vi "RTS Get TDMS Data.vi"(0 "CSV Data Save":T2, 1 "Chamber 1 Socket":string[][](array[string]), 2 "Chamber 2 Socket":string[][](array[string]), 3 "Chamber 3 Socket":string[][](array[string]), 4 "Chamber 4 Socket":string[][](array[string]), 5 "error in (no error)":errorcluster, 9 "Tree Selection":T1) -> (14 "Station Data":dbl[][](array[numeric]), 15 "Point File Name":string, 19 "error out":errorcluster)   [LabVIEW 2016]
uses:
  Type Definitions/RTS TDMS Filename Locations.ctl
  Type Definitions/RTS Save References.ctl
  Type Definitions/RTS Room Selector.ctl
  Type Definitions/RTS TDMS Data.ctl
panel:
  out "Indexed Full Names":string[](array[string])
  out "Index Locations":i32[](array[numeric])
  out "Custom Titles":string[](array[string])
  out "Item Names":string[](array[string])
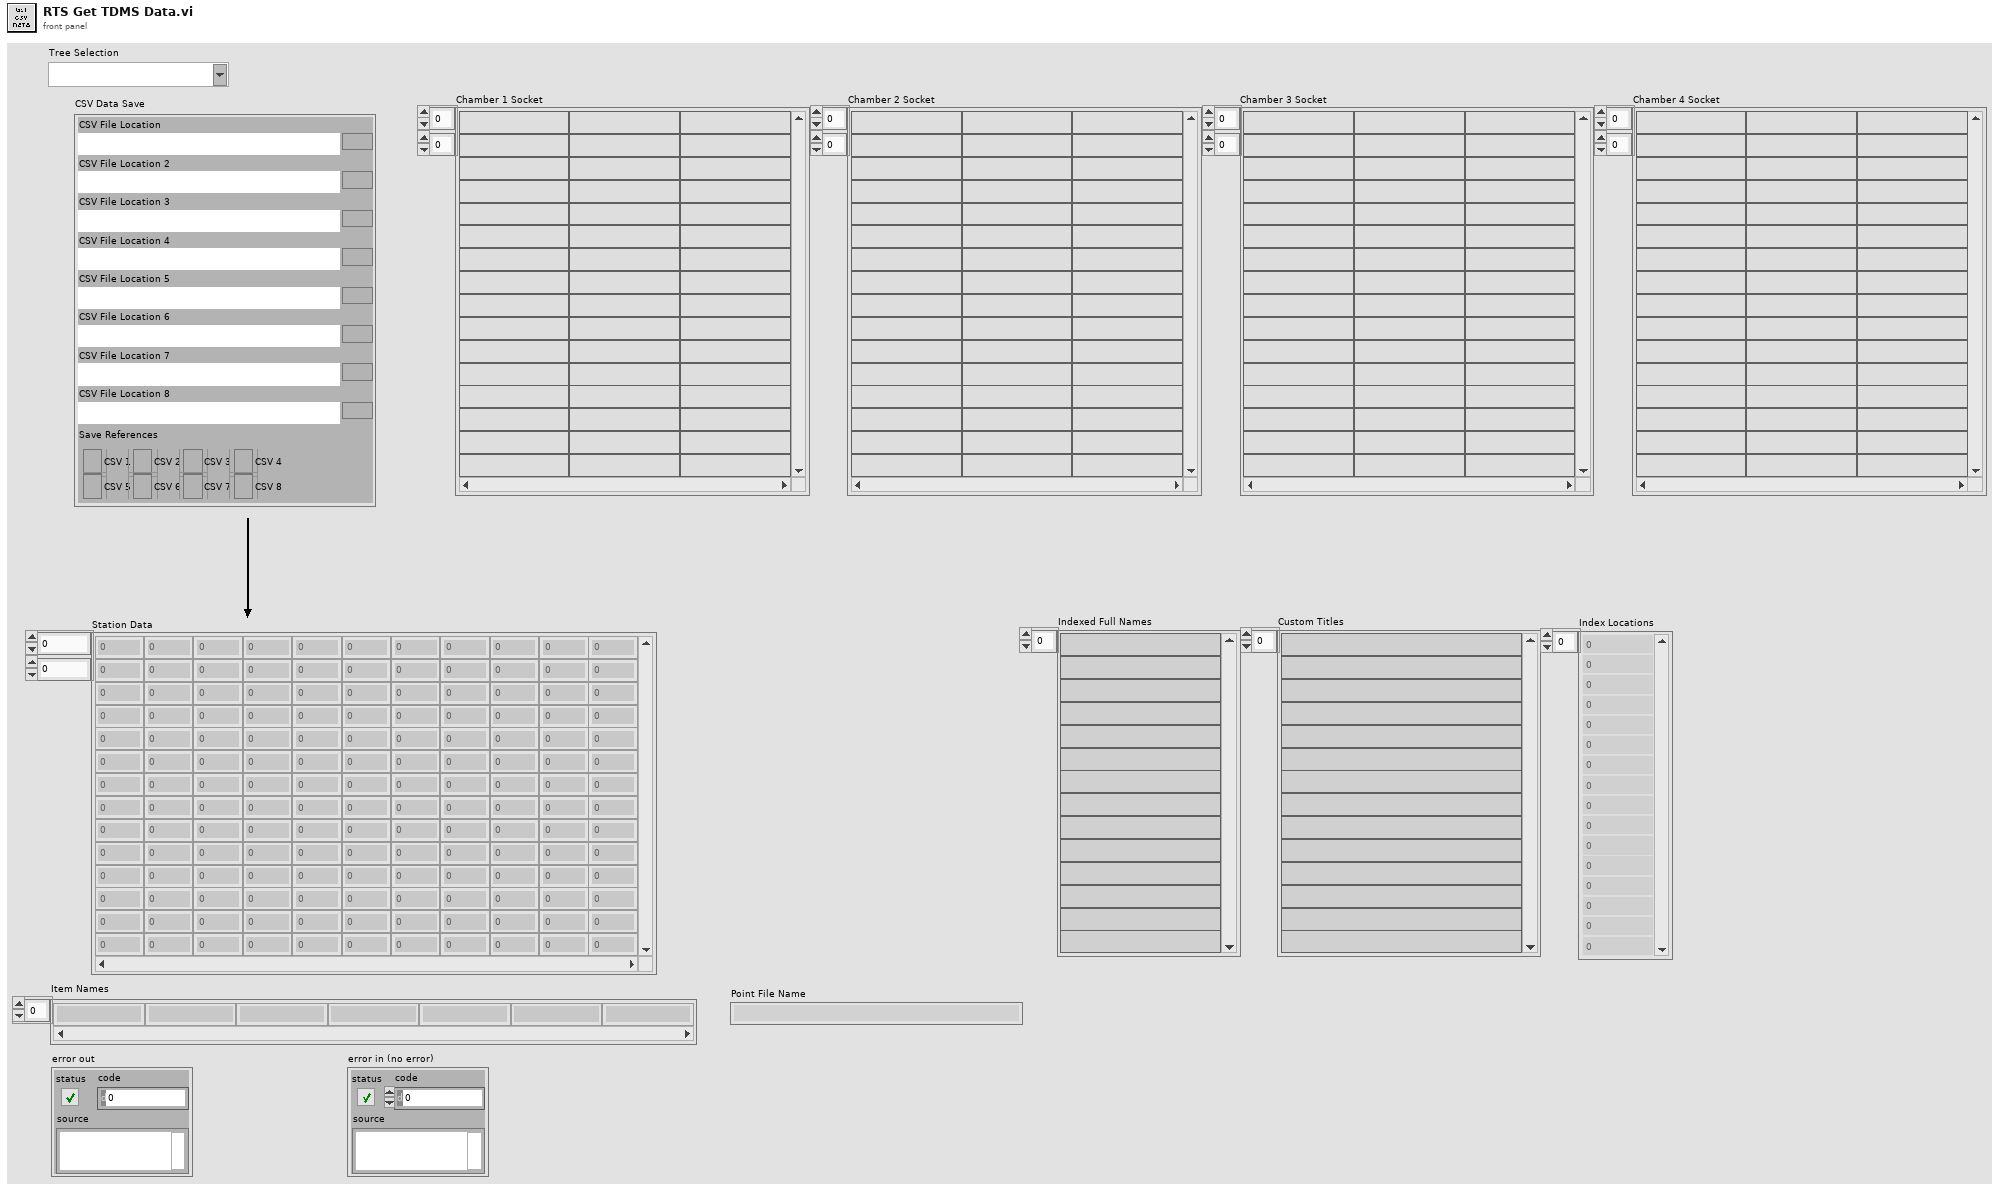
[diagram p1: front panel]
types:
  T1 = typedef "RTS Room Selector.ctl" = string
  T2 = typedef "RTS TDMS Filename Locations.ctl" = cluster{"CSV File Location":path, "CSV File Location 2":path, "CSV File Location 3":path, "CSV File Location 4":path, "CSV File Location 5":path, "CSV File Location 6":path, "CSV File Location 7":path, "CSV File Location 8":path, "Save References":T3}
  T3 = typedef "RTS Save References.ctl" = cluster{"CSV 1":refnum<file>, "CSV 2":refnum<file>, "CSV 3":refnum<file>, "CSV 4":refnum<file>, "CSV 5":refnum<file>, "CSV 6":refnum<file>, "CSV 7":refnum<file>, "CSV 8":refnum<file>}
  T4 = typedef "RTS TDMS Data.ctl" = cluster{"Station 1":dbl[][], "Station 2":dbl[][], "Station 3":dbl[][], "Station 4":dbl[][], "Station 5":dbl[][], "Station 6":dbl[][], "Station 7":dbl[][], "Station 8":dbl[][]}
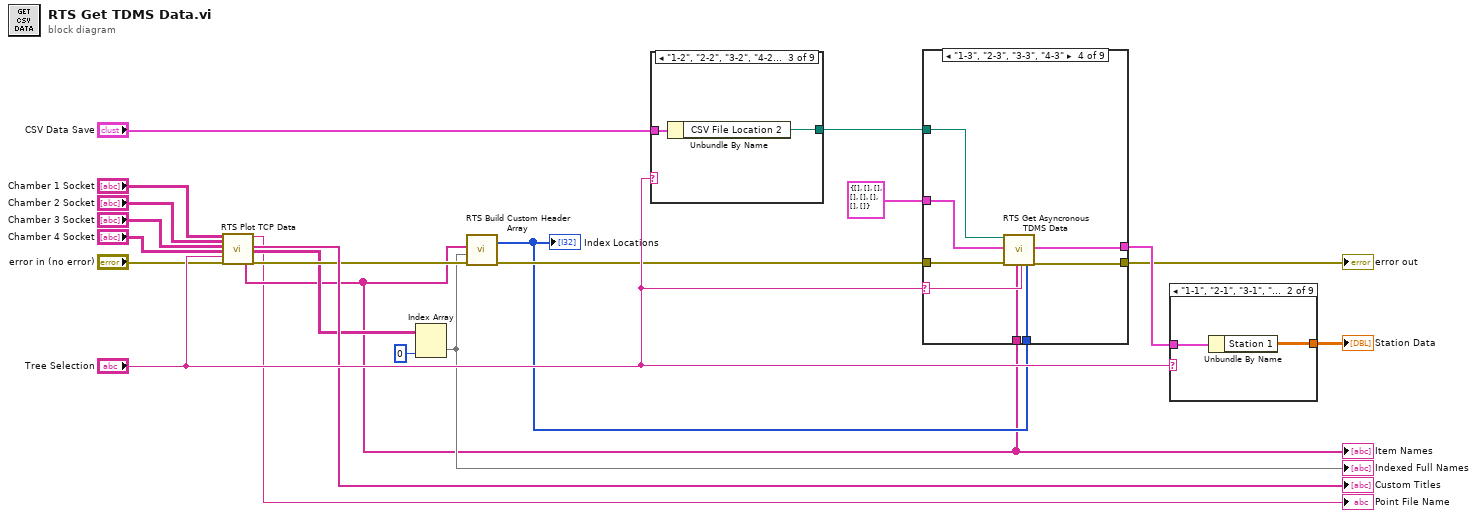
[diagram p0: block diagram]
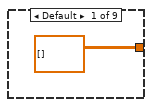
[diagram p2: hidden frame]
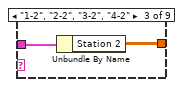
[diagram p3: hidden frame]
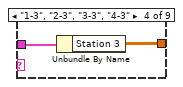
[diagram p4: hidden frame]
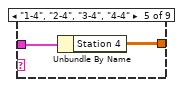
[diagram p5: hidden frame]
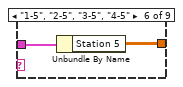
[diagram p6: hidden frame]
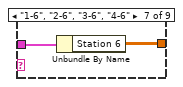
[diagram p7: hidden frame]
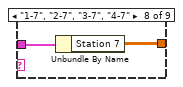
[diagram p8: hidden frame]
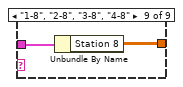
[diagram p9: hidden frame]
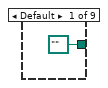
[diagram p10: hidden frame]
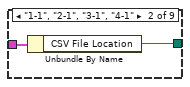
[diagram p11: hidden frame]
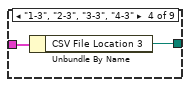
[diagram p12: hidden frame]
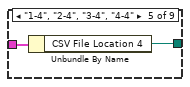
[diagram p13: hidden frame]
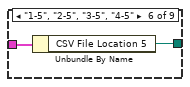
[diagram p14: hidden frame]
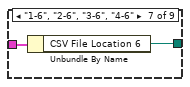
[diagram p15: hidden frame]
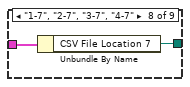
[diagram p16: hidden frame]
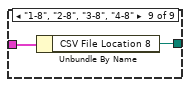
[diagram p17: hidden frame]
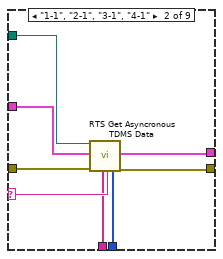
[diagram p19: hidden frame]
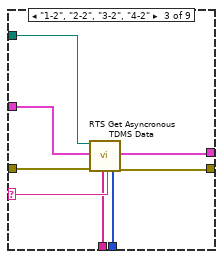
[diagram p20: hidden frame]
diagram:
  n1 = call "RTS Plot TCP Data.vi"("Chamber 1 Socket"="Chamber 1 Socket", "Chamber 2 Socket"="Chamber 2 Socket", "Chamber 3 Socket"="Chamber 3 Socket", "Chamber 4 Socket"="Chamber 4 Socket", "Tree Selection in"="Tree Selection", "Error In"="error in (no error)") -> ("Full Item Names"=w3:string[], "Point File Name"=→"Point File Name":string, "Custom Titles"=→"Custom Titles":string[], "Listbox Data"=w11:string[][], "Error Out"=w13:errorcluster)  [unwired: 6 in, 3 out]
  "Item Names" <- w3
  n2 = Index Array(array=w11, index (col)=0 ("disabled index (col)")) -> (element=w9:string[])  [unwired: 1 in]
  "Indexed Full Names" <- w9
  n3 = call "RTS Build Custom Header Array.vi"("Error In"=w13, "Listbox Item Names in"=w9, "Full Item Names"=w3) -> ("Error Out"=w12:errorcluster, "Index Locations"=w4:i32[])  [unwired: 4 in, 3 out]
  "Index Locations" <- w4
  n4 = case shown="\"1-2\", \"2-2\", \"3-2\", \"4-2\"" "Tree Selection" {
    tunnel: "CSV Data Save" -> [_ w24 w26 w28 w30 w32 w34 w36 w38]
    tunnel: [path "" ("CSV File Location 7") w23 w25 w27 w29 w31 w33 w35 w37] -> w7
    frame Default {
    }
    frame "1-1", "2-1", "3-1", "4-1" {
      n5 = Unbundle By Name(w24) -> ("CSV File Location"=w23:path)
    }
    frame "1-2", "2-2", "3-2", "4-2" {
      n6 = Unbundle By Name(w26) -> ("CSV File Location 2"=w25:path)
    }
    frame "1-3", "2-3", "3-3", "4-3" {
      n7 = Unbundle By Name(w28) -> ("CSV File Location 3"=w27:path)
    }
    frame "1-4", "2-4", "3-4", "4-4" {
      n8 = Unbundle By Name(w30) -> ("CSV File Location 4"=w29:path)
    }
    frame "1-5", "2-5", "3-5", "4-5" {
      n9 = Unbundle By Name(w32) -> ("CSV File Location 5"=w31:path)
    }
    frame "1-6", "2-6", "3-6", "4-6" {
      n10 = Unbundle By Name(w34) -> ("CSV File Location 6"=w33:path)
    }
    frame "1-7", "2-7", "3-7", "4-7" {
      n11 = Unbundle By Name(w36) -> ("CSV File Location 7"=w35:path)
    }
    frame "1-8", "2-8", "3-8", "4-8" {
      n12 = Unbundle By Name(w38) -> ("CSV File Location 8"=w37:path)
    }
  }
  n13 = case shown="\"1-3\", \"2-3\", \"3-3\", \"4-3\"" "Tree Selection" {
    selector: "Tree Selection" -> [_ w43 w51 w59 w67 w76 w85 w92 w101]
    tunnel: T4 {"Station 1"=[], "Station 2"=[], "Station 3"=[], "Station 4"=[], "Station 5"=[], "Station 6"=[], "Station 7"=[], "Station 8"=[]} ("CSV Data") -> [w39 w48 w54 w62 w70 w79 w87 w95 w99]
    tunnel: [w39 w47 w55 w63 w71 w75 w83 w91 w104] -> w6
    tunnel: w7 -> [_ w46 w56 w64 w72 w80 w88 w96 w100]
    tunnel: w12 -> [w40 w45 w53 w61 w69 w78 w86 w94 w102]
    tunnel: [w40 w44 w52 w60 w68 w77 w84 w93 w103] -> w1
    tunnel: w4 -> [_ w42 w49 w57 w65 w73 w81 w89 w97]
    tunnel: w3 -> [_ w41 w50 w58 w66 w74 w82 w90 w98]
    frame Default {
    }
    frame "1-1", "2-1", "3-1", "4-1" {
      n14 = call "RTS Get Asyncronous TDMS Data.vi"("File Location"=w46, "CVS Data Input"=w48, "error in (no error)"=w45, "Full Item Names"=w41, "Station ID"=w43, "Index Locations"=w42) -> ("CVS Data Output"=w47:T4, "error out"=w44:errorcluster)  [unwired: 12 in]
    }
    frame "1-2", "2-2", "3-2", "4-2" {
      n15 = call "RTS Get Asyncronous TDMS Data.vi"("File Location"=w56, "CVS Data Input"=w54, "error in (no error)"=w53, "Full Item Names"=w50, "Station ID"=w51, "Index Locations"=w49) -> ("CVS Data Output"=w55:T4, "error out"=w52:errorcluster)  [unwired: 12 in]
    }
    frame "1-3", "2-3", "3-3", "4-3" {
      n16 = call "RTS Get Asyncronous TDMS Data.vi"("File Location"=w64, "CVS Data Input"=w62, "error in (no error)"=w61, "Full Item Names"=w58, "Station ID"=w59, "Index Locations"=w57) -> ("CVS Data Output"=w63:T4, "error out"=w60:errorcluster)  [unwired: 12 in]
    }
    frame "1-4", "2-4", "3-4", "4-4" {
      n17 = call "RTS Get Asyncronous TDMS Data.vi"("File Location"=w72, "CVS Data Input"=w70, "error in (no error)"=w69, "Full Item Names"=w66, "Station ID"=w67, "Index Locations"=w65) -> ("CVS Data Output"=w71:T4, "error out"=w68:errorcluster)  [unwired: 12 in]
    }
    frame "1-5", "2-5", "3-5", "4-5" {
      n18 = call "RTS Get Asyncronous TDMS Data.vi"("File Location"=w80, "CVS Data Input"=w79, "error in (no error)"=w78, "Full Item Names"=w74, "Station ID"=w76, "Index Locations"=w73) -> ("CVS Data Output"=w75:T4, "error out"=w77:errorcluster)  [unwired: 12 in]
    }
    frame "1-6", "2-6", "3-6", "4-6" {
      n19 = call "RTS Get Asyncronous TDMS Data.vi"("File Location"=w88, "CVS Data Input"=w87, "error in (no error)"=w86, "Full Item Names"=w82, "Station ID"=w85, "Index Locations"=w81) -> ("CVS Data Output"=w83:T4, "error out"=w84:errorcluster)  [unwired: 12 in]
    }
    frame "1-7", "2-7", "3-7", "4-7" {
      n20 = call "RTS Get Asyncronous TDMS Data.vi"("File Location"=w96, "CVS Data Input"=w95, "error in (no error)"=w94, "Full Item Names"=w90, "Station ID"=w92, "Index Locations"=w89) -> ("CVS Data Output"=w91:T4, "error out"=w93:errorcluster)  [unwired: 12 in]
    }
    frame "1-8", "2-8", "3-8", "4-8" {
      n21 = call "RTS Get Asyncronous TDMS Data.vi"("File Location"=w100, "CVS Data Input"=w99, "error in (no error)"=w102, "Full Item Names"=w98, "Station ID"=w101, "Index Locations"=w97) -> ("CVS Data Output"=w104:T4, "error out"=w103:errorcluster)  [unwired: 12 in]
    }
  }
  "error out" <- w1
  n22 = case shown="\"1-1\", \"2-1\", \"3-1\", \"4-1\"" "Tree Selection" {
    tunnel: [dbl[][] [] w107 w109 w111 w113 w115 w117 w119 w121] -> w5
    tunnel: w6 -> [_ w106 w108 w110 w112 w114 w116 w118 w120]
    frame Default {
    }
    frame "1-1", "2-1", "3-1", "4-1" {
      n23 = Unbundle By Name(w106) -> ("Station 1"=w107:dbl[][])
    }
    frame "1-2", "2-2", "3-2", "4-2" {
      n24 = Unbundle By Name(w108) -> ("Station 2"=w109:dbl[][])
    }
    frame "1-3", "2-3", "3-3", "4-3" {
      n25 = Unbundle By Name(w110) -> ("Station 3"=w111:dbl[][])
    }
    frame "1-4", "2-4", "3-4", "4-4" {
      n26 = Unbundle By Name(w112) -> ("Station 4"=w113:dbl[][])
    }
    frame "1-5", "2-5", "3-5", "4-5" {
      n27 = Unbundle By Name(w114) -> ("Station 5"=w115:dbl[][])
    }
    frame "1-6", "2-6", "3-6", "4-6" {
      n28 = Unbundle By Name(w116) -> ("Station 6"=w117:dbl[][])
    }
    frame "1-7", "2-7", "3-7", "4-7" {
      n29 = Unbundle By Name(w118) -> ("Station 7"=w119:dbl[][])
    }
    frame "1-8", "2-8", "3-8", "4-8" {
      n30 = Unbundle By Name(w120) -> ("Station 8"=w121:dbl[][])
    }
  }
  "Station Data" <- w5
